vi "SetMode Test.vi"(8 "Error In":errorcluster, 11 "WiFi Server Mode":T1(ring)=enum."WIFI_AP") -> (0 "Error Out":errorcluster)   [LabVIEW 2014, in "ESP8266 WiFi Wrapper.lvlib"]
uses:
  <vilib>/Aledyne-TSXperts/Arduino Compatible Compiler for LabVIEW/addons/ESP8266 WiFi Wrapper/ESP8266 WiFi Wrapper.lvlib
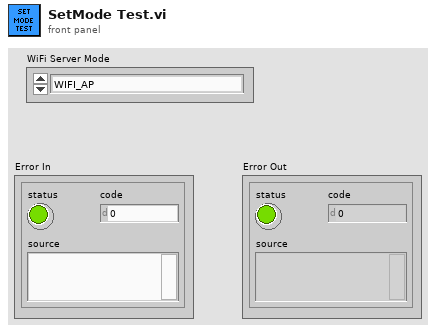
[diagram p1: front panel]
types:
  T1 = enum16{"WIFI_OFF", "WIFI_STA", "WIFI_AP", "WIFI_AP_STA"}
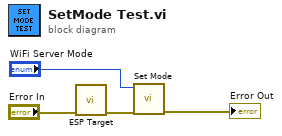
[diagram p0: block diagram]
diagram:
  n1 = call <vilib>:"ESP Target.vi"("Error In"="Error In") -> ("Error Out"=w1:errorcluster)  [unwired: 10 in]
  n2 = call <vilib>:"Set Mode.vi"("Error In"=w1, "WiFi Server Mode"="WiFi Server Mode") -> ("Error Out"=→"Error Out":errorcluster)  [unwired: 9 in]
